vi "Filter Tips.vi"(8 "error in (no error)":errorcluster, 10 "Duplicate Distance":dbl, 11 "Tips":T1[](array[typedef]) {"ROI Descriptor"."Contours"."Type" items=["No Selection", "Point", "Line", "Rectangle", "Oval", "Polygon", "Freehand Region", "Annulus", "Unused2", "Unused3", "Broken Line", "Freehand Line", "Rotated Rectangle"]; "Point"."Y" format="%.2f"; "Point"."X" format="%.2f"}) -> (0 "error out":errorcluster, 3 "Filtered Tips":T1[](array[typedef]) {"ROI Descriptor"."Contours"."Type" items=["No Selection", "Point", "Line", "Rectangle", "Oval", "Polygon", "Freehand Region", "Annulus", "Unused2", "Unused3", "Broken Line", "Freehand Line", "Rotated Rectangle"]; "Point"."Y" format="%.2f"; "Point"."X" format="%.2f"})   [LabVIEW 2013]
uses:
  Controls/Tip.ctl
  <vilib>/vision/NI_Vision_Development_Module.lvlib
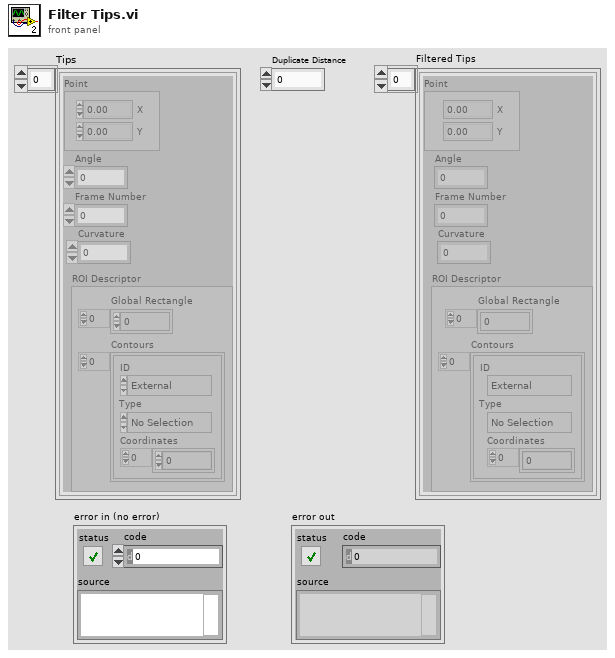
[diagram p1: front panel]
types:
  T1 = typedef "Tip.ctl" = cluster{"Point":T2, "Angle":dbl, "Frame Number":i32, "ROI Descriptor":T3, "Curvature":dbl}
  T2 = typedef "IMAQ Point" = cluster{"X":sgl, "Y":sgl}
  T3 = typedef "ROI Descriptor" = cluster{"Global Rectangle":i32[], "Contours":cluster{"ID":enum32{"External", "Internal"}, "Type":u32, "Coordinates":i32[]}[]}
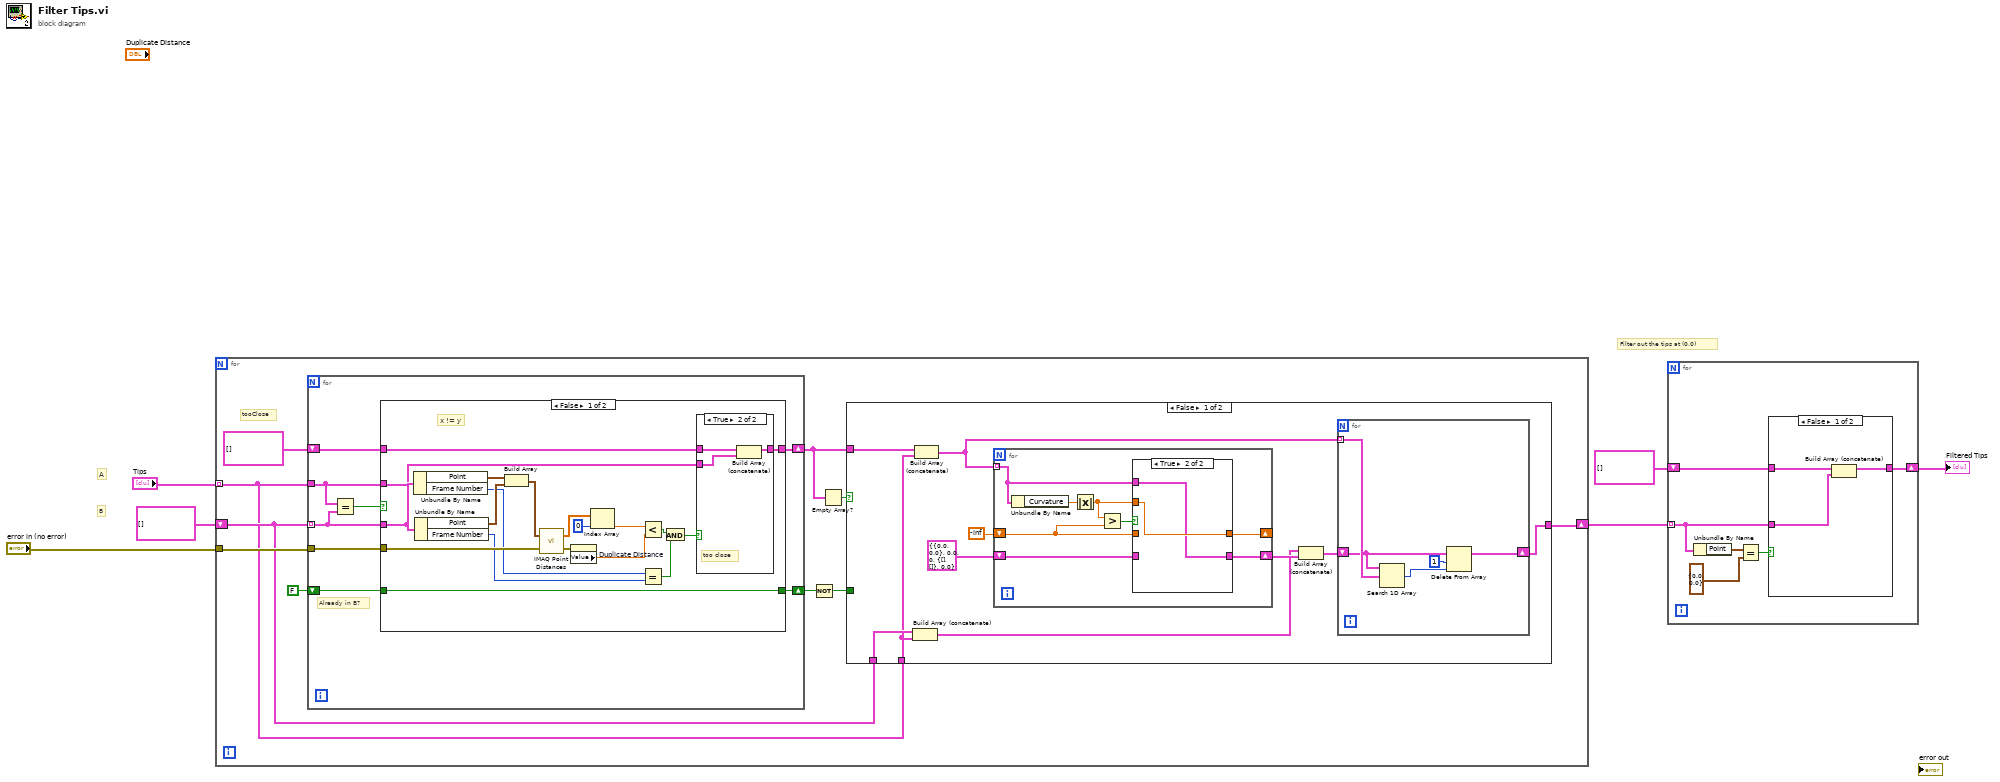
[diagram p0: block diagram]
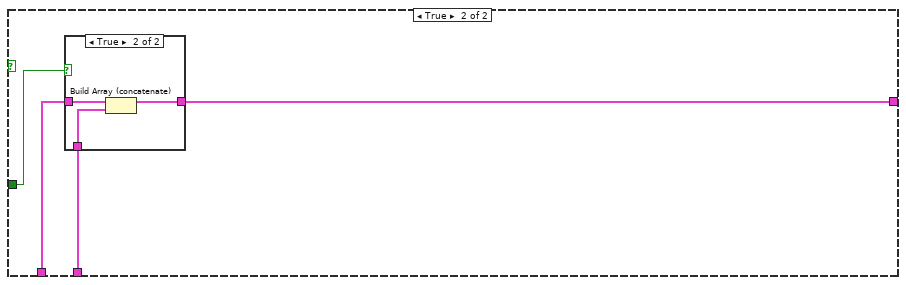
[diagram p4: hidden frame]
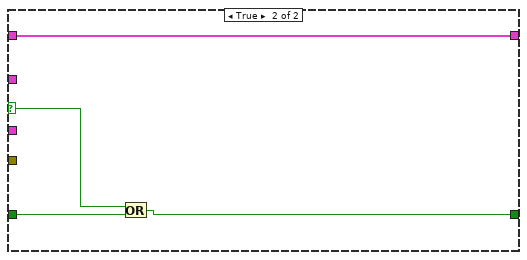
[diagram p7: hidden frame]
diagram:
  # "Filter out the tips at (0,0)"
  # "B"
  # "A"
  n1 = for {
    tunnel: "Tips" -> [w11] mode=indexing
    shift-right: [w8] -> w3
    shift-left: T1[] [] ("appended array") -> [w12]
    tunnel: "error in (no error)" -> [w14]
    # "tooClose"
    n2 = for {
      tunnel: w12 -> [w54] mode=indexing
      shift-right: [w57] -> w13
      shift-left: FALSE -> [w58]
      tunnel: w11 -> [w55]
      shift-right: [w52] -> w7
      shift-left: T1[] [] ("appended array") -> [w56]
      tunnel: w14 -> [w53]
      # "Already in B?"
      n3 = Equal?(x=w55, y=w54) -> (x = y?=w59:bool)
      n4 = case shown="False" w59 {
        selector: w59 -> [_ w85]
        tunnel: w58 -> [w78 w86]
        tunnel: [w78 w84] -> w57
        tunnel: w56 -> [w68 w83]
        tunnel: w55 -> [w67 _]
        tunnel: w54 -> [w66 _]
        tunnel: w53 -> [w69 _]
        tunnel: [w65 w83] -> w52
        frame False {
          # "x != y"
          n5 = Unbundle By Name(w67) -> ("Point"=w70:T2, "Frame Number"=w61:i32)
          n6 = Unbundle By Name(w66) -> ("Point"=w71:T2, "Frame Number"=w60:i32)
          n7 = Build Array(w70, w71) -> (w72:T2[])
          n8 = call "IMAQ Point Distances"("Points"=w72, "error in (no error)"=w69) -> ("Distances"=w73:sgl[], "error out"=w76:errorcluster)  [unwired: 3 in]
          n9 = property on="Duplicate Distance" class="DigNum (strict)"(error in=w76) -> ("Value"=w77:dbl)  [unwired: 1 in, 2 out]
          n10 = Index Array(array=w73, index=0) -> (element=w75:sgl)
          n11 = Less?(x=w75, y=w77) -> (x < y?=w64:bool)
          n12 = Equal?(x=w61, y=w60) -> (x = y?=w62:bool)
          n13 = And(x=w64, y=w62) -> (x .and. y?=w63:bool)
          n14 = case shown="True" w63 {
            tunnel: w68 -> [w79 w82]
            tunnel: w66 -> [_ w81]
            tunnel: [w79 w80] -> w65
            frame False {
            }
            frame True {
              # "too close"
              n15 = Build Array (concatenate)(w82, w81) -> (w80:T1[])
            }
          }
        }
        frame True {
          n16 = Or(x=w85, y=w86) -> (x .or. y?=w84:bool)
        }
      }
    }
    n17 = Not(x=w13) -> (.not. x?=w9:bool)
    n18 = Empty Array?(array=w7) -> (empty?=w10:bool)
    n19 = case shown="False" w10 {
      tunnel: w12 -> [w25 w47]
      tunnel: w11 -> [w23 w46]
      tunnel: w9 -> [_ w45]
      tunnel: [w17 w44] -> w8
      tunnel: w7 -> [w26 _]
      frame False {
        n20 = Build Array (concatenate)(w25, w23) -> (w20:T1[])
        n21 = Build Array (concatenate)(w26, w23) -> (w18:T1[])
        n22 = for {
          tunnel: w18 -> [w32] mode=indexing
          shift-right: [w35] -> _
          shift-left: -inf -> [w36]
          shift-right: [w34] -> w21
          shift-left: T1 {"Point"={"X"=0.0, "Y"=0.0}, "Angle"=0.0, "Frame Number"=0, "ROI Descriptor"={"Global Rectangle"=[], "Contours"=[]}, "Curvature"=0.0} ("Tip") -> [w33]
          n23 = Unbundle By Name(w32) -> ("Curvature"=w39:dbl)
          n24 = Absolute Value(x=w39) -> (abs(x)=w37:dbl)
          n25 = Greater?(x=w37, y=w36) -> (0:w38:bool)
          n26 = case shown="True" w38 {
            tunnel: w37 -> [_ w43]
            tunnel: w36 -> [w41 _]
            tunnel: [w41 w43] -> w35
            tunnel: [w40 w42] -> w34
            tunnel: w33 -> [w40 _]
            tunnel: w32 -> [_ w42]
            frame False {
            }
            frame True {
            }
          }
        }
        n27 = Build Array (concatenate)(w20, w21) -> (w19:T1[])
        n28 = for {
          shift-right: [w29] -> w17
          shift-left: w19 -> [w30]
          tunnel: w18 -> [w31] mode=indexing
          n29 = Search 1D Array(1D array=w30, element=w31) -> (index of element=w28:i32)  [unwired: 1 in]
          n30 = Delete From Array(array=w30, length=1, index=w28) -> (array with subset deleted=w29:T1[])  [unwired: 1 out]
        }
      }
      frame True {
        n31 = case shown="True" w45 {
          tunnel: w47 -> [w48 w51]
          tunnel: [w48 w50] -> w44
          tunnel: w46 -> [_ w49]
          frame False {
          }
          frame True {
            n32 = Build Array (concatenate)(w51, w49) -> (w50:T1[])
          }
        }
      }
    }
  }
  n33 = for {
    tunnel: w3 -> [w87] mode=indexing
    shift-right: [w88] -> w1
    shift-left: T1[] [] ("appended array") -> [w89]
    n34 = Unbundle By Name(w87) -> ("Point"=w92:T2)
    n35 = Equal?(x=w92, y=T2 {"X"=0.0, "Y"=0.0} ("Point")) -> (x = y?=w90:bool)
    n36 = case shown="False" w90 {
      tunnel: w89 -> [w95 w96]
      tunnel: [w94 w96] -> w88
      tunnel: w87 -> [w93 _]
      frame False {
        n37 = Build Array (concatenate)(w95, w93) -> (w94:T1[])
      }
      frame True {
      }
    }
  }
  "Filtered Tips" <- w1
